vi "Normal Log.vi"(8 "error in (no error)":errorcluster, 10 "log":string, 11 "Normal Log in":refnum<class "Normal Log.lvclass">) -> (0 "error out":errorcluster, 3 "Normal Log out":refnum<class "Normal Log.lvclass">)   [LabVIEW 2020, in "Normal Log.lvlib" / "Normal Log.lvclass"]
uses:
  Normal Log.lvclass
  Normal Log Messages/Append Log List Msg/Append Log List Msg.lvclass
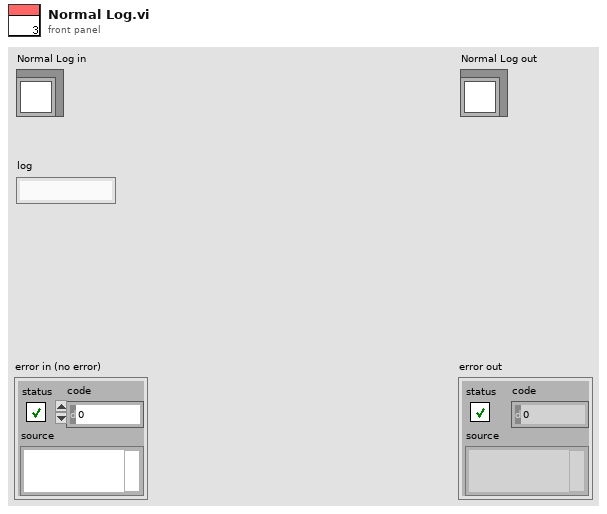
[diagram p1: front panel]
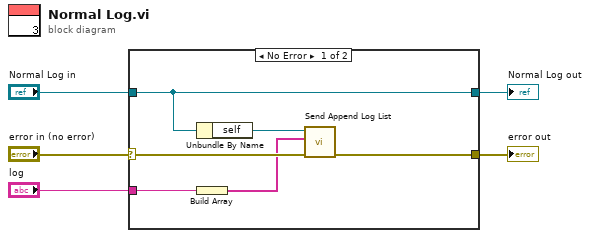
[diagram p0: block diagram]
diagram:
  n1 = case shown="No Error" "error in (no error)" {
    selector: "error in (no error)" -> [w10 w13]
    tunnel: "log" -> [w7 _]
    tunnel: "Normal Log in" -> [w11 w12]
    tunnel: [w9 w13] -> w2
    tunnel: [w11 w12] -> w1
    frame No Error {
      n2 = Unbundle By Name(w11) -> ("self"=w8:refnum<class "Message Enqueuer.lvclass">)
      n3 = Build Array(w7) -> (w6:string[])
      n4 = call "Send Append Log List.vi"("error in (no error)"=w10, "log list"=w6, "Message Enqueuer"=w8) -> ("error out"=w9:errorcluster)  [unwired: 7 in, 1 out]
    }
    frame Error {
    }
  }
  "error out" <- w2
  "Normal Log out" <- w1
